vi "FTW-CSV-Escape.vi"(1 "String":string) -> (0 "Escaped UTF-8 String":string)   [LabVIEW 2015]
panel:
  # "Inputs"
  # "Outputs"
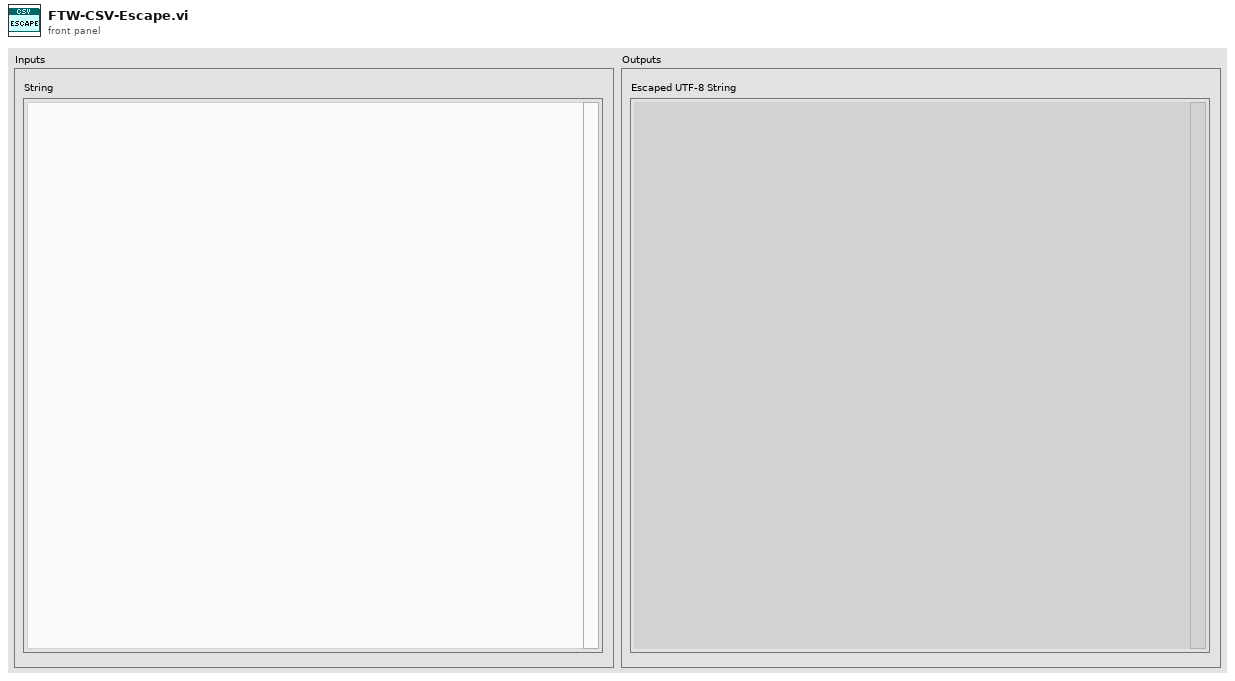
[diagram p1: front panel]
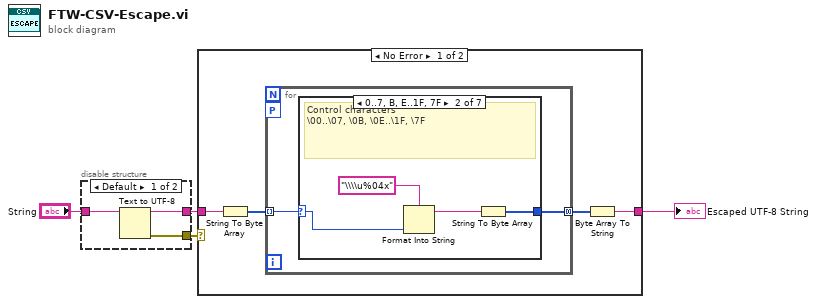
[diagram p0: block diagram]
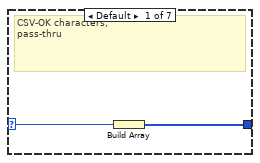
[diagram p3: hidden frame]
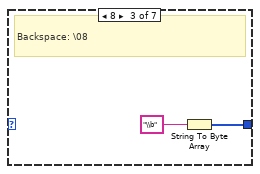
[diagram p4: hidden frame]
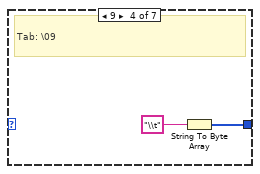
[diagram p5: hidden frame]
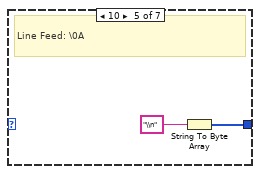
[diagram p6: hidden frame]
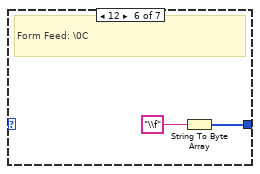
[diagram p7: hidden frame]
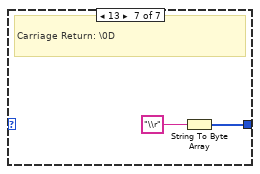
[diagram p8: hidden frame]
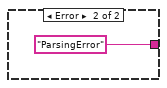
[diagram p9: hidden frame]
diagram:
  n1 = disable-structure shown="Default" {
    disable-tunnel: "String" -> [w7 w8]
    disable-tunnel: [w6 w8] -> w2
    disable-tunnel: [w5 _] -> w1
    frame condition #0 (active) {
      n2 = Text to UTF-8(11:w7) -> (0:w5:errorcluster, 3:w6:string)  [unwired: 2 in]
    }
    frame condition #1 {
    }
  }
  n3 = case shown="No Error" w1 {
    tunnel: [w11 "ParsingError" ("Escaped String")] -> w4
    tunnel: w2 -> [w10 _]
    frame No Error {
      n4 = String To Byte Array(string=w10) -> (unsigned byte array=w9:u8[])
      n5 = for {
        tunnel: [w14] -> w12 mode=concatenating
        tunnel: w9 -> [w13] mode=indexing
        workers-P: _ -> [_]
        n6 = case shown="0..7, B, E..1F, 7F" w13 {
          selector: w13 -> [w16 w18 _ _ _ _ _]
          tunnel: [w15 w17 w21 w23 w25 w27 w29] -> w14
          frame Default {
            # "CSV-OK characters;\npass-thru"
            n7 = Build Array(w16) -> (w15:u8[])
          }
          frame 0..7, 11, 14..31, 127 {
            # "Control characters\n\\00..\\07, \\0B, \\0E..\\1F, \\7F"
            n8 = Format Into String(format string="\\\\u%04x", w18) -> (resulting string=w19:string)  [unwired: 2 in, 1 out]
            n9 = String To Byte Array(string=w19) -> (unsigned byte array=w17:u8[])
          }
          frame 8 {
            # "Backspace: \\08"
            n10 = String To Byte Array(string="\\b") -> (unsigned byte array=w21:u8[])
          }
          frame 9 {
            # "Tab: \\09"
            n11 = String To Byte Array(string="\\t") -> (unsigned byte array=w23:u8[])
          }
          frame 10 {
            # "Line Feed: \\0A"
            n12 = String To Byte Array(string="\\n") -> (unsigned byte array=w25:u8[])
          }
          frame 12 {
            # "Form Feed: \\0C"
            n13 = String To Byte Array(string="\\f") -> (unsigned byte array=w27:u8[])
          }
          frame 13 {
            # "Carriage Return: \\0D"
            n14 = String To Byte Array(string="\\r") -> (unsigned byte array=w29:u8[])
          }
        }
      }
      n15 = Byte Array To String(unsigned byte array=w12) -> (string=w11:string)
    }
    frame Error {
    }
  }
  "Escaped UTF-8 String" <- w4
